vi "serialInit.vi"(6 "timeout":dbl=0.01, 8 "error in (no error)":errorcluster, 9 "Baud":u32=115200, 10 "Port":string, 11 "Python":T1) -> (0 "error out":errorcluster, 2 "port name":string, 3 "Processor":T2)   [LabVIEW 2022 SP3]
uses:
  Processors.ctl
  PythonCtrl.ctl
  <vilib>/Instr/_visa.llb/VISA Configure Serial Port (Instr).vi
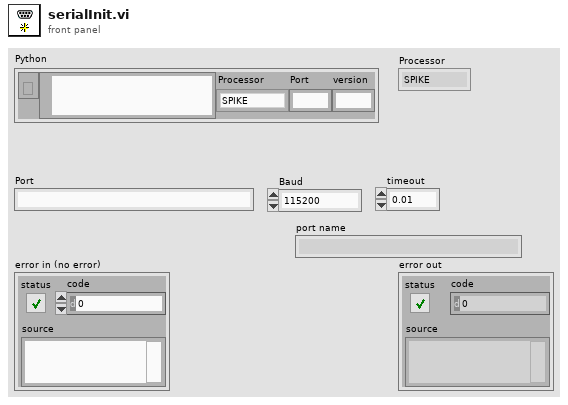
[diagram p1: front panel]
types:
  T1 = typedef "PythonCtrl.ctl" = cluster{"session":refnum<k35>, "PyPath":path, "Processor":T2, "Port":string, "version":string}
  T2 = typedef "Processors.ctl" = enum16{"SPIKE", "Pi", "Pi_ssh", "OpenMV", "Dunio"}
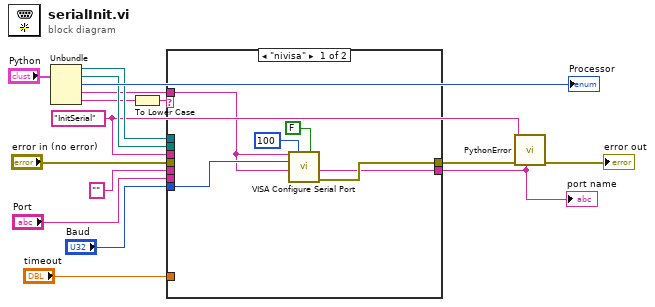
[diagram p0: block diagram]
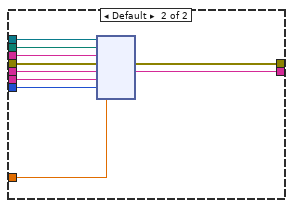
[diagram p2: hidden frame]
diagram:
  w4 = "InitSerial" ("function name")
  n1 = Unbundle("Python") -> ("session"=w13:refnum<k35>, "PyPath"=w12:path, "Processor"=→"Processor":T2, "Port"=w1:string, "version"=w3:string)
  n2 = To Lower Case(string=w3) -> (all lower case string=w2:string)
  n3 = case shown="\"nivisa\"" w2 {
    tunnel: "" ("function name") -> [_ w31]
    tunnel: "Baud" -> [w21 w30]
    tunnel: w13 -> [_ w29]
    tunnel: w12 -> [_ w28]
    tunnel: "Port" -> [_ w27]
    tunnel: "error in (no error)" -> [_ w26]
    tunnel: "timeout" -> [_ w25]
    tunnel: [w19 w24] -> w7
    tunnel: [w18 w23] -> w5
    tunnel: w4 -> [_ w22]
    tunnel: w1 -> [w18 _]
    frame "nivisa" {
      n4 = call-poly "VISA Configure Serial Port"("VISA resource name"=w18, "timeout (10sec)"=u32 100, "Enable Termination\nChar (T)"=FALSE ("Enable Termination\nChar (T)"), "baud rate (9600)"=w21) -> ("error out"=w19:errorcluster)  [unwired: 10 in, 1 out]
    }
    frame Default {
      n5 = node(w29, w28, w22, w26, w31, w27, w30, w25) -> (w24:errorcluster, w23:string)  [unwired: 3 in, 3 out]
    }
  }
  "port name" <- w5
  n6 = call "PythonError.vi"("reply"=w5, "error in (no error)"=w7, "function name"=w4) -> ("error out"=→"error out":errorcluster)  [unwired: 8 in]
